vi "SubPanel Main.vi"() -> ()   [LabVIEW 2015]
panel:
  in  "Listbox":i32(listbox)
  in  "Fill Listbox":bool
  in  "Stop Button":bool
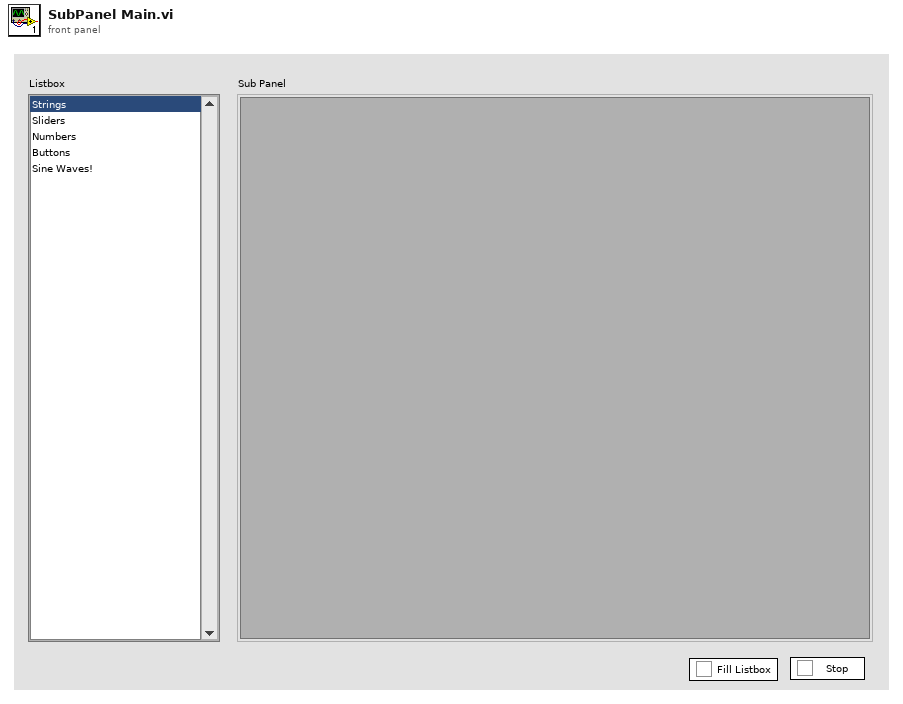
[diagram p1: front panel]
types:
  T1 = enum16{"Always On", "Always Off", "Off While Running"}
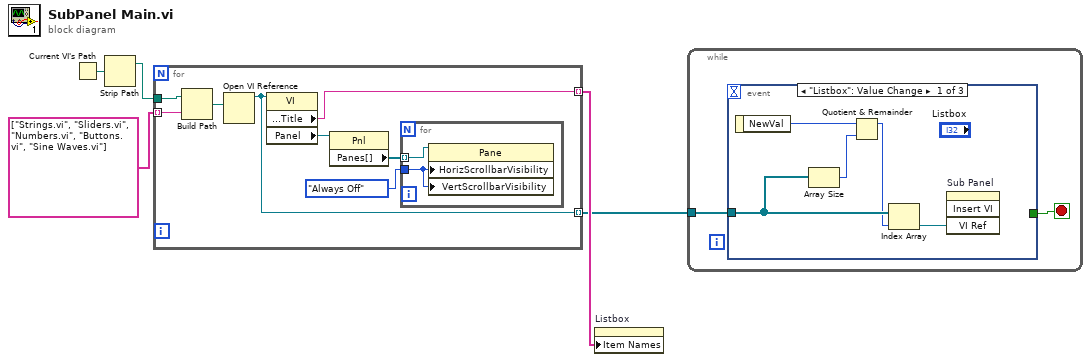
[diagram p0: block diagram]
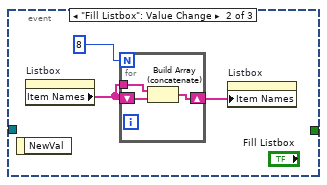
[diagram p2: hidden frame]
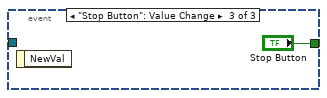
[diagram p3: hidden frame]
diagram:
  n1 = Current VI's Path() -> (path=w2:path)
  n2 = Strip Path(path=w2) -> (stripped path=w1:path)  [unwired: 1 out]
  n3 = for {
    tunnel: string[] ["Strings.vi", "Sliders.vi", "Numbers.vi", "Buttons.vi", "Sine Waves.vi"] -> [w11] mode=indexing
    tunnel: [w13] -> w3 mode=indexing
    tunnel: [w12] -> w4 mode=indexing
    tunnel: w1 -> [w10]
    n4 = Build Path(base path=w10, name or relative path=w11) -> (appended path=w9:path)
    n5 = Open VI Reference(vi path=w9) -> (vi reference=w13:refnum<vi>)  [unwired: 5 in, 1 out]
    n6 = property class="VI"(reference=w13) -> ("Front Panel.Title"=w12:string, "Panel"=w8:refnum<vi>)  [unwired: 1 in, 2 out]
    n7 = property class="Pnl"(reference=w8) -> ("Panes[]"=w7:refnum<vi>[])  [unwired: 1 in, 2 out]
    n8 = for {
      tunnel: w7 -> [w15] mode=indexing
      tunnel: T1."Always Off" ("Horizontal Scrollbar Visibility") -> [w14]
      n9 = property class="Pane"(reference=w15, "HorizScrollbarVisibility"=w14, "VertScrollbarVisibility"=w14) -> ()  [unwired: 1 in, 2 out]
    }
  }
  n10 = property on="Listbox" class="LstBox (strict)"("Item Names"=w4) -> ()  [unwired: 2 in, 2 out]
  n11 = while {
    tunnel: w3 -> [w17]
    stop <- w16 stop-if-true
    n12 = event shown="[0] \"Listbox\": Value Change" {
      selector: _ -> [_ _ _]
      dyn-events: _ -> [_ _ _]
      timeout: _ -> [_ _ _]
      tunnel: w17 -> [w19 _ _]
      tunnel: [_ _ "Stop Button"] -> w16
      event "Listbox": Value Change {
        n13 = event-data() -> ("NewVal"=w20:i32)  [unwired: 1 in]
        n14 = Array Size(array=w19) -> (size(s)=w21:i32)
        n15 = Quotient & Remainder(x=w20, y=w21) -> (x-y*floor(x/y)=w18:i32)  [unwired: 1 out]
        n16 = Index Array(array=w19, index=w18) -> (element=w22:refnum<vi>)
        n17 = invoke on="Sub Panel" class="SubPanel" method="Insert VI"("VI Ref"=w22) -> ()  [unwired: 3 in, 4 out]
      }
      event "Fill Listbox": Value Change {
        n18 = event-data() -> ()  [unwired: 1 in, 1 out]
        n19 = property on="Listbox" class="LstBox (strict)"() -> ("Item Names"=w25:string[])  [unwired: 2 in, 2 out]
        n20 = for {
          N: 8 -> [_]
          tunnel: w25 -> [w28]
          shift-right: [w27] -> w24
          shift-left: w25 -> [w26]
          n21 = Build Array (concatenate)(w28, w26) -> (w27:string[])
        }
        n22 = property on="Listbox" class="LstBox (strict)"("Item Names"=w24) -> ()  [unwired: 2 in, 2 out]
      }
      event "Stop Button": Value Change {
        n23 = event-data() -> ()  [unwired: 1 in, 1 out]
      }
    }
  }
